vi "Float to Modbus.vi"(10 "32-Bit Float":sgl) -> (2 "Registers":u16[](array[numeric]) format="%016b")   [LabVIEW 2024, in "Bronkhorst Flexi-Flow ModbusTCP API.lvlib"]
uses:
  Bronkhorst Flexi-Flow ModbusTCP API.lvlib
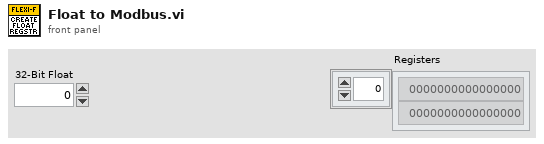
[diagram p1: front panel]
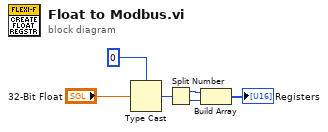
[diagram p0: block diagram]
diagram:
  n1 = Type Cast(type=u32 0, x="32-Bit Float") -> (*(type *) &x=w4:u32)
  n2 = Split Number(x=w4) -> (hi(x)=w2:u16, lo(x)=w3:u16)
  n3 = Build Array(w2, w3) -> (→"Registers":u16[])
